vi "Configure Serial Bus (SENT - Source).vi"(0 "VISA resource name":refnum<visa-resource-name>, 1 "Nibble Length (1)":i32=1, 2 "Idle State (0: Low)":u16(ring) items=["Low", "High"], 5 "Serial Bus Name (1: Serial Bus 1)":u16(ring)=1 items=["Serial Bus 1"=1, "Serial Bus 2"=2], 7 "Clock Period (1 micro sec)":dbl=1.0, 9 "Tolerance (3%)":i32=3, 11 "error in (no error)":errorcluster, 12 "CRC Format (0: Recommended)":u16(ring) items=["Recommended (2010)", "Legacy (2008)"], 13 "Enable Pause Pulse  (False:)":bool) -> (4 "VISA resource name out":refnum<visa-resource-name>, 15 "error out":errorcluster)   [LabVIEW 2015, in "Agilent 2000 3000 X-Series.lvlib"]
doc: "Configures SENT signal source parameters."
uses:
  <instrlib>/Agilent 2000 3000 X-Series/Agilent 2000 3000 X-Series.lvlib
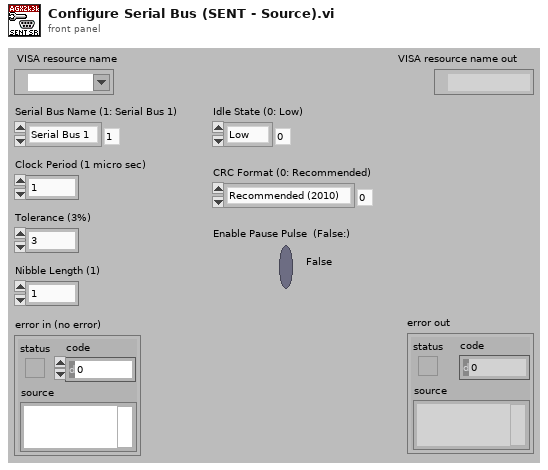
[diagram p1: front panel]
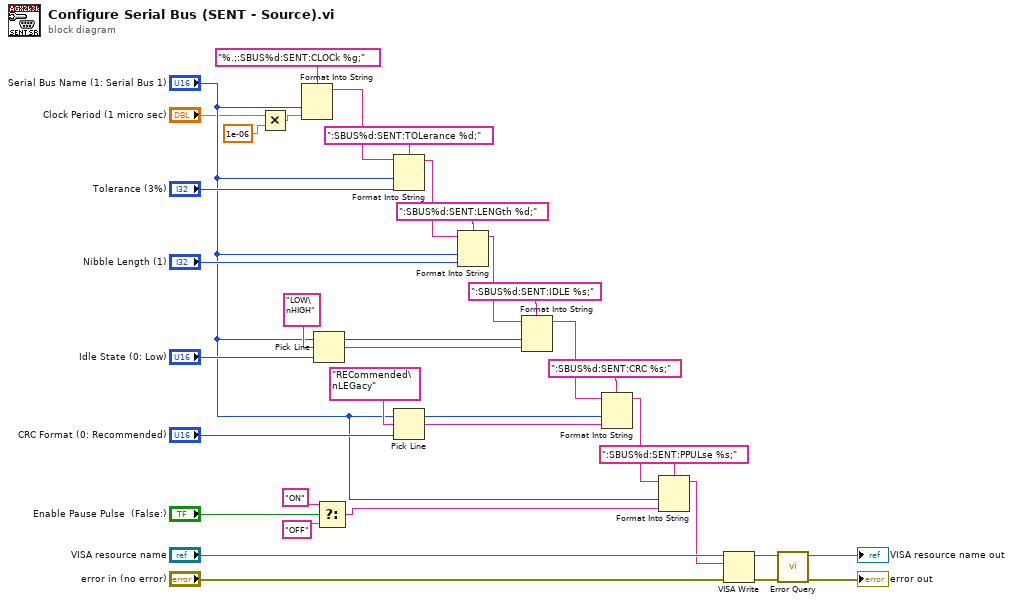
[diagram p0: block diagram]
diagram:
  n1 = Multiply(x="Clock Period (1 micro sec)", y=1e-06) -> (x*y=w2:dbl)
  n2 = Format Into String(format string="%.;:SBUS%d:SENT:CLOCk %g;", "Serial Bus Name (1: Serial Bus 1)", w2) -> (resulting string=w31:string)  [unwired: 2 in, 1 out]
  n3 = Pick Line(multi-line string="LOW\nHIGH", line index="Idle State (0: Low)") -> (output string=w24:string)  [unwired: 1 in]
  n4 = Select(t="ON", s="Enable Pause Pulse  (False:)", f="OFF") -> (s? t:f=w16:string)
  n5 = Format Into String(format string=":SBUS%d:SENT:TOLerance %d;", initial string=w31, "Serial Bus Name (1: Serial Bus 1)", "Tolerance (3%)") -> (resulting string=w28:string)  [unwired: 1 in, 1 out]
  n6 = Pick Line(multi-line string="RECommended\nLEGacy", line index="CRC Format (0: Recommended)") -> (output string=w23:string)  [unwired: 1 in]
  n7 = Format Into String(format string=":SBUS%d:SENT:LENGth %d;", initial string=w28, "Serial Bus Name (1: Serial Bus 1)", "Nibble Length (1)") -> (resulting string=w11:string)  [unwired: 1 in, 1 out]
  n8 = Format Into String(format string=":SBUS%d:SENT:IDLE %s;", initial string=w11, "Serial Bus Name (1: Serial Bus 1)", w24) -> (resulting string=w10:string)  [unwired: 1 in, 1 out]
  n9 = Format Into String(format string=":SBUS%d:SENT:CRC %s;", initial string=w10, "Serial Bus Name (1: Serial Bus 1)", w23) -> (resulting string=w9:string)  [unwired: 1 in, 1 out]
  n10 = Format Into String(format string=":SBUS%d:SENT:PPULse %s;", initial string=w9, "Serial Bus Name (1: Serial Bus 1)", w16) -> (resulting string=w8:string)  [unwired: 1 in, 1 out]
  n11 = VISA Write(VISA resource name="VISA resource name", write buffer=w8, error in (no error)="error in (no error)") -> (VISA resource name out=w7:refnum<visa-resource-name>, error out=w6:errorcluster)  [unwired: 1 out]
  n12 = call <instrlib>:"Error Query.vi"("error in (no error)"=w6, "VISA resource name"=w7) -> ("error out"=→"error out":errorcluster, "VISA resource name out"=→"VISA resource name out":refnum<visa-resource-name>)  [unwired: 6 in, 2 out]
